vi "Configure Voltage Parameters.vi"(0 "Session Handle in":T6, 11 "error in (no error)":errorcluster) -> (4 "Session Handle out":T6, 15 "error out":errorcluster)   [LabVIEW 2019, in "SmartScopeDriver.lvclass"]
doc: "Configures the Voltage Sensitivity and Signal Setup Parameters."
uses:
  SmartScopeDriver.lvclass
  Typedefs/Session Handle.ctl
  Scope Driver/Typedef/Vertical Settings.ctl
  Scope Driver/Typedef/Channel Selection.ctl
  Scope Driver/Typedef/Coupling.ctl
  Scope Driver/Typedef/RangeSetting.ctl
  Scope Driver/Typedef/Metadata/[Meta]SetupInfoV.ctl
  SmartScopeDriver.lvclass/SmartScopeDriver.ctl
  Scope Driver/LabNation Scope Driver.lvlib
panel:
  out "[Meta]SetupInfoV":T1
  in  "Vertical Settings":T3={"ChannelSelection"=enum."chn A", "Coupling"=0, "Offset[V]"=0.0, "V/div"=4.0} {"V/div" scale=0.0..6.0; "Coupling" items=["AC", "DC"]}
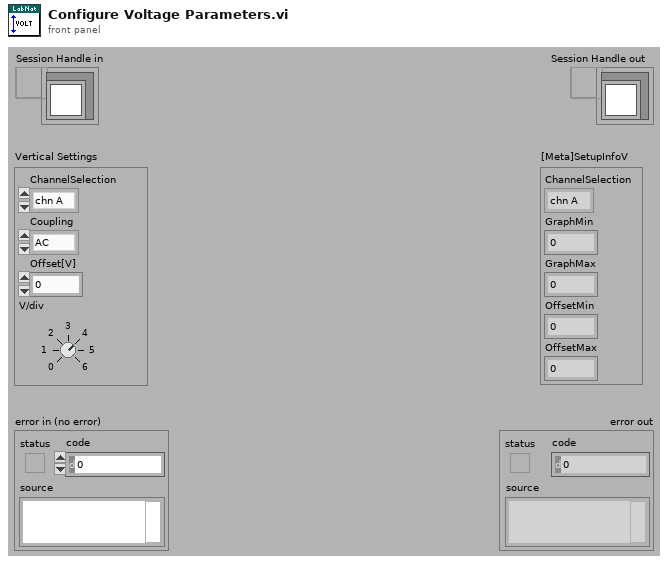
[diagram p1: front panel]
types:
  T1 = typedef "LabNation Scope Driver.lvlib/[Meta]SetupInfoV.ctl" = cluster{"ChannelSelection":T2, "GraphMin":dbl, "GraphMax":dbl, "OffsetMin":dbl, "OffsetMax":dbl}
  T2 = typedef "LabNation Scope Driver.lvlib/Channel Selection.ctl" = enum16{"chn A", "chn B"}
  T3 = typedef "LabNation Scope Driver.lvlib/Vertical Settings.ctl" = cluster{"ChannelSelection":T2, "Coupling":T4, "Offset[V]":dbl, "V/div":T5}
  T4 = typedef "LabNation Scope Driver.lvlib/Coupling.ctl" = i32
  T5 = typedef "LabNation Scope Driver.lvlib/RangeSetting.ctl" = dbl
  T6 = typedef "SmartScopeDriver.lvclass/Session Handle.ctl" = refnum<data-value>
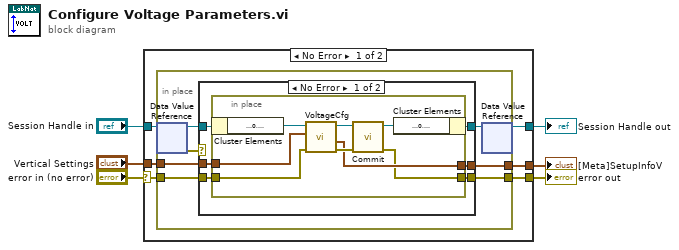
[diagram p0: block diagram]
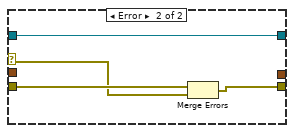
[diagram p2: hidden frame]
diagram:
  n1 = case shown="No Error" "error in (no error)" {
    selector: "error in (no error)" -> [w10 w38]
    tunnel: "Session Handle in" -> [w12 w39]
    tunnel: [w11 w39] -> w5
    tunnel: [w9 w38] -> w4
    tunnel: [w8 _] -> w2
    tunnel: "Vertical Settings" -> [w7 _]
    frame No Error {
      n2 = in-place {
        in-place-border: w10 -> [w15]
        in-place-border: [w18] -> w9
        in-place-border: [w14] -> w8
        in-place-border: w7 -> [w13]
        n3 = in-place-dvr #1(w12) -> (w19:refnum<class "SmartScopeDriver.lvclass">, w16:errorcluster)
        n4 = case shown="No Error" w16 {
          selector: w16 -> [_ w36]
          tunnel: w19 -> [w25 w34]
          tunnel: [w24 w35] -> w18
          tunnel: [w23 w34] -> w17
          tunnel: w15 -> [w22 w37]
          tunnel: [w21 _] -> w14
          tunnel: w13 -> [w20 _]
          frame No Error {
            n5 = in-place {
              in-place-border: [w28] -> w24
              in-place-border: w22 -> [w32]
              in-place-border: [w30] -> w21
              in-place-border: w20 -> [w29]
              n6 = in-place-cluster #2(w25) -> ("reference"=w33:refnum<k24>)
              n7 = call "VoltageCfg.vi"("error in (no error)"=w32, "Vertical Settings"=w29, "reference in"=w33) -> ("error out"=w31:errorcluster, "[Meta]SetupInfoV"=w30:T1, "reference out"=w27:refnum<k24>)  [unwired: 6 in]
              n8 = call "Commit.vi"("error in (no error)"=w31, "reference in"=w27) -> ("error out"=w28:errorcluster, "reference out"=w26:refnum<k24>)  [unwired: 8 in]
              n9 = in-place-cluster #2("reference"=w26) -> (w23:refnum<class "SmartScopeDriver.lvclass">)
            }
          }
          frame Error {
            n10 = Merge Errors(w37, w36) -> (w35:errorcluster)
          }
        }
        n11 = in-place-dvr #1(w17) -> (w11:T6)  [unwired: 1 out]
      }
    }
    frame Error {
    }
  }
  "Session Handle out" <- w5
  "error out" <- w4
  "[Meta]SetupInfoV" <- w2
